vi "OpenScan LabVIEW Host.vi"() -> ()   [LabVIEW 2015]
uses:
  <vilib>/FPGAPlugInAG/PXIe-7972R/niLvFpga_Open_PXIe-7972R.vi
  <vilib>/rvi/interface/common/dynamic/niFpgaDynamicAddResources.vi
  <vilib>/FPGAPlugInAG/Dynamic/niLvFpga_Reset_Dynamic.vi
  <vilib>/FPGAPlugInAG/Dynamic/niLvFpga_Run_Dynamic.vi
  <vilib>/Utility/error.llb/Error Cluster From Error Code.vi
  <vilib>/rvi/errors/niLvFpgaAdjustHostInterfaceError.vi
  <vilib>/rvi/interface/nirviOpenFPGA/nirviOpenFPGA.xnode
  FPGA Bitfiles/OpenScan_FPGATarget_OpenScanFPGAHost_IYDpsE60iho.lvbitx
  OpenScan LabVIEW FPGA/OpenScan FPGA Host.vi
  <vilib>/rvi/interface/nirviMethod/nirviMethod.xnode
  <vilib>/rvi/interface/nirviReadWriteControl/nirviReadWriteControl.xnode
  <vilib>/rvi/interface/Simulation/niFpgaSimulationCallBeginRW.vi
  NiFpgaLv.dll
  <vilib>/rvi/errors/niLvFpgaMergeErrorWithErrorCode.vi
  <vilib>/FPGAPlugInAG/Dynamic/niLvFpga_ReadFifo_Dynamic.vi
  <vilib>/FPGAPlugInAG/Dynamic/niLvFpga_WriteFifo_Dynamic.vi
  <vilib>/FPGAPlugInAG/Dynamic/niLvFpga_StopFifo_Dynamic.vi
panel:
  out "error out":errorcluster
  out "Frame Galvo signal write done?":bool
  out "Total elements 2":u32
  out "Get status":bool=TRUE
  out "max addr":u32
  out "Ready to scan":bool
  out "Ready to initialize FPGA":bool
  in  "Filter gain":fxp<+,16,0>=0.9999847412109375 format="%.16g"
  out "Kalman done":u32
  out "Kalman done?":bool
  out "Galvo Y":u16[][](graph)
  out "Galvo X":u16[][](graph)
  out "Frames done":i32
  out "Original Image":T1(plugin-control)
  out "Kalman averaged image":T1(plugin-control)
  out "Blank image data":u32[](array[numeric])
  out "Averaged image displayed?":bool
  in  "Kalman averaging factor":u32=1
  in  "Num of frames":i32=214758367
  in  "Imaging mode":i16(ring)=2 items=["Grab, single frame", "Loop, finite frames", "Focus, infinite frames"]
  in  "Pixel clock_pulse width ratio":dbl=0.8 format="%#_13g"
  in  "Scan rate":dbl=0.25 format="%#_13g"
  in  "ZoomY":dbl=0.8 step=0.1
  in  "Zoom X":sgl=0.8 step=0.1
  in  "Calculate parameters":bool caption="停止"
  in  "Max DRAM address":u32
  in  "Frame number":i32
  in  "Samples per frame control":u32
  in  "Frame retrace time(ms)":u32=100
  in  "Number of frames":i32
  in  "Pixel pulse_initial delay":i32=1
  in  "Pixel clock_pulse width(tick)":i32
  in  "Resolution":i32(ring)=512 items=["2048"=2048, "1024"=1024, "512"=512, "256"=256]
  in  "Num of undershoot":i32=50
  in  "Elements per line":i32=1000
  in  "Total elements":u32
  in  "Pixel time (tick)":i32
  out "Image averaging done?":bool
  out "Frame acquisition done":bool
  out "Frame waveform output done":bool
  out "Waveform written to DRAM":bool
  out "Current status":T2(ring)
  in  "stop":bool caption="停止"
  in  "Load Waveform":bool caption="元素入队列"
  in  "Start Scanning":bool caption="元素入队列"
  in  "Initialize FPGA":bool caption="停止"
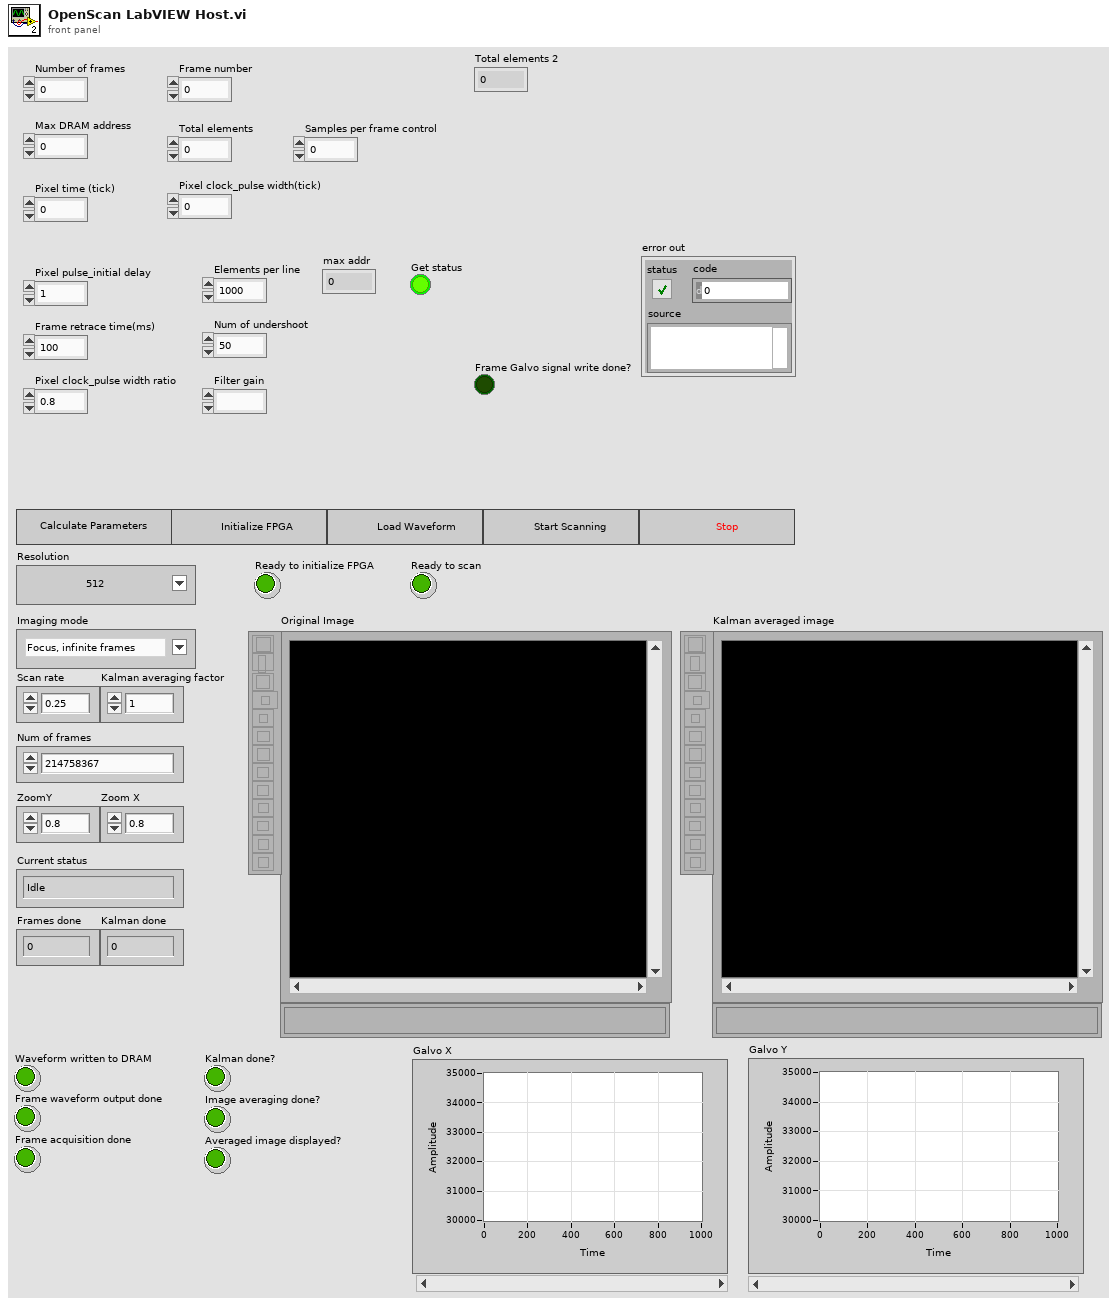
[diagram p1: front panel]
types:
  T1 = typedef "IMAQ Image.ctl" = refnum<image>
  T2 = enum16{"Idle", "Init", "Write", "Scan", "Blank", "Stop"}
  T3 = enum8{"Enabled", "Disabled", "Disabled and Grayed Out"}
  T4 = typedef "Image Type" = u32
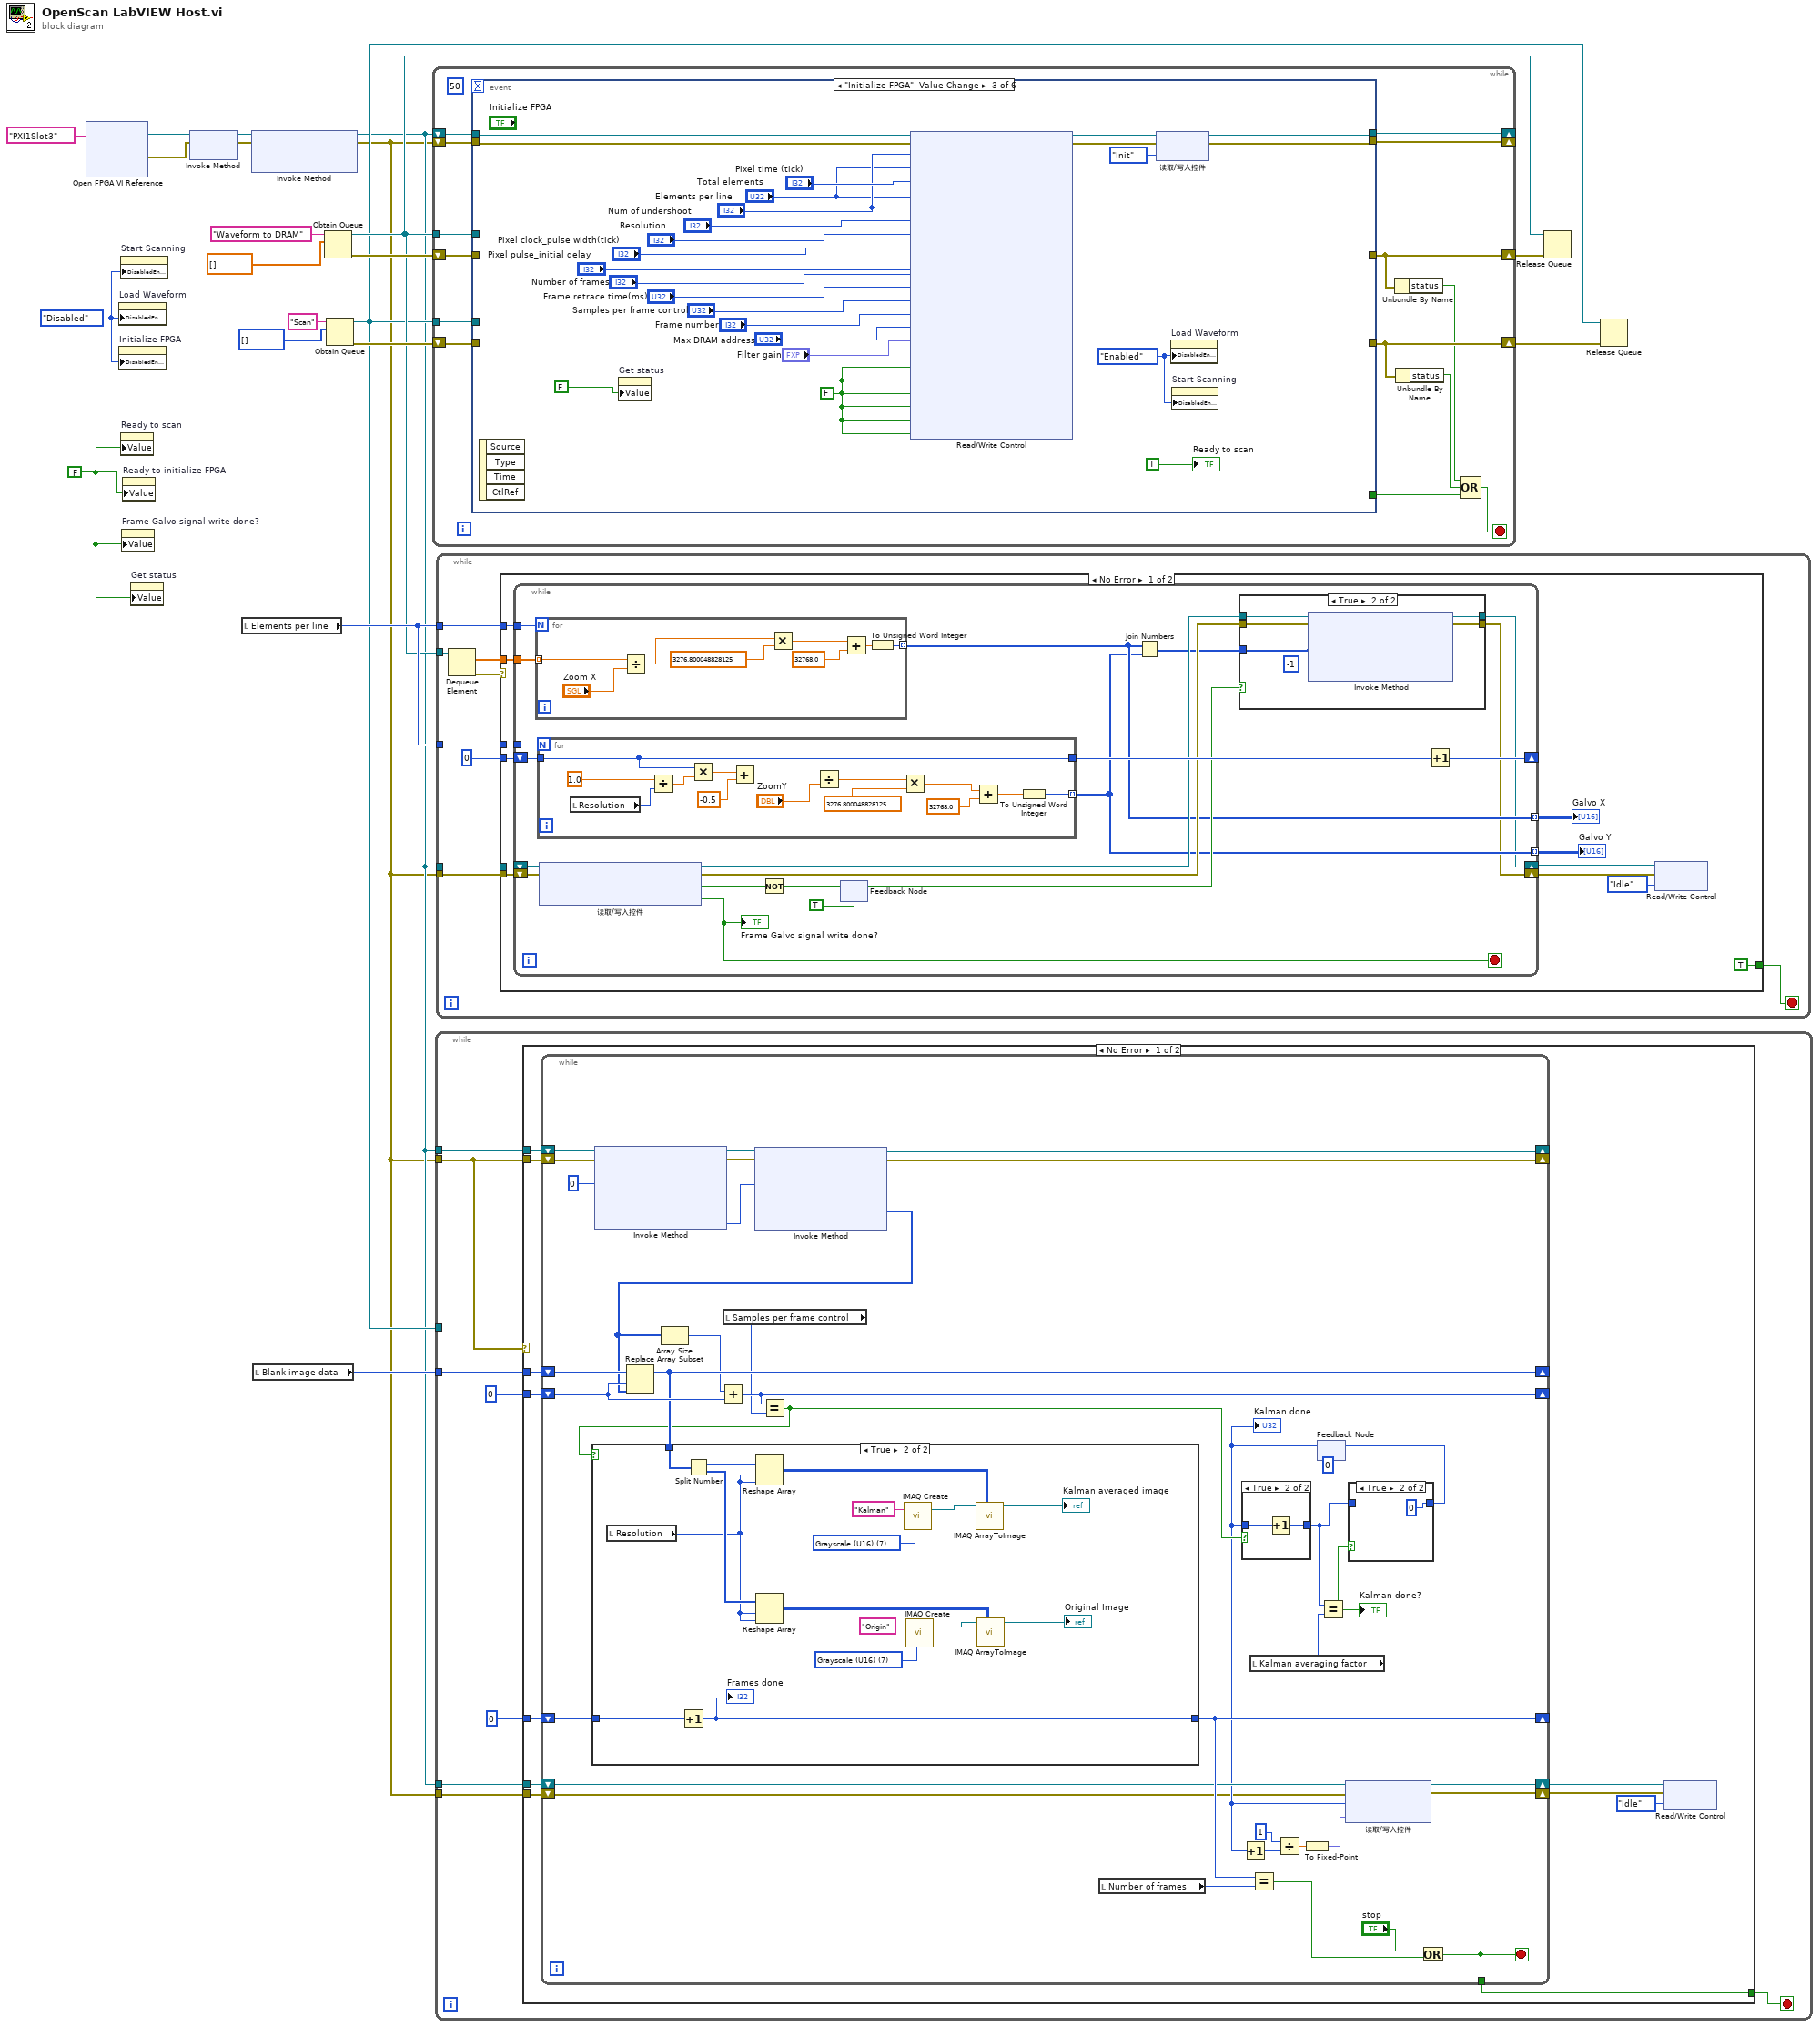
[diagram p0: block diagram]
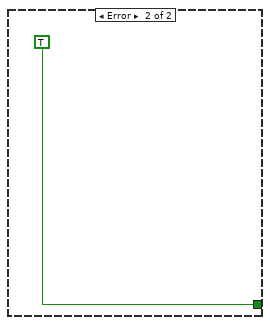
[diagram p5: hidden frame]
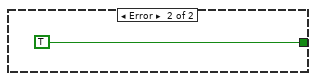
[diagram p7: hidden frame]
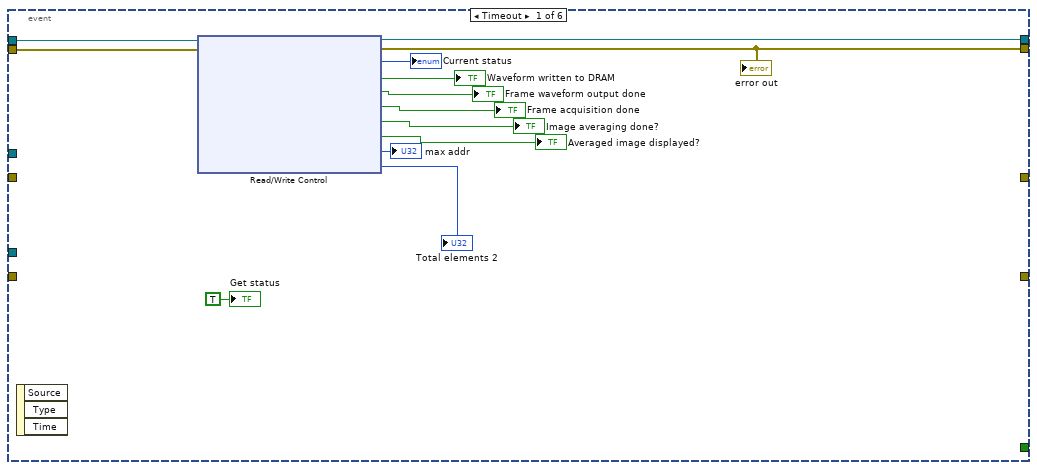
[diagram p8: hidden frame]
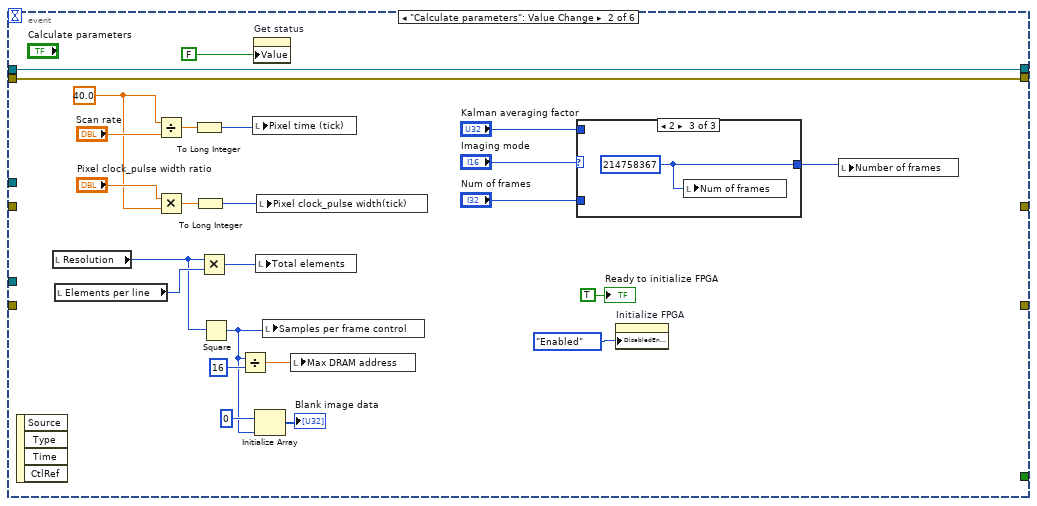
[diagram p9: hidden frame]
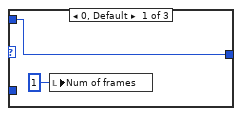
[diagram p10: hidden frame]
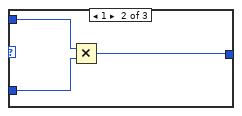
[diagram p11: hidden frame]
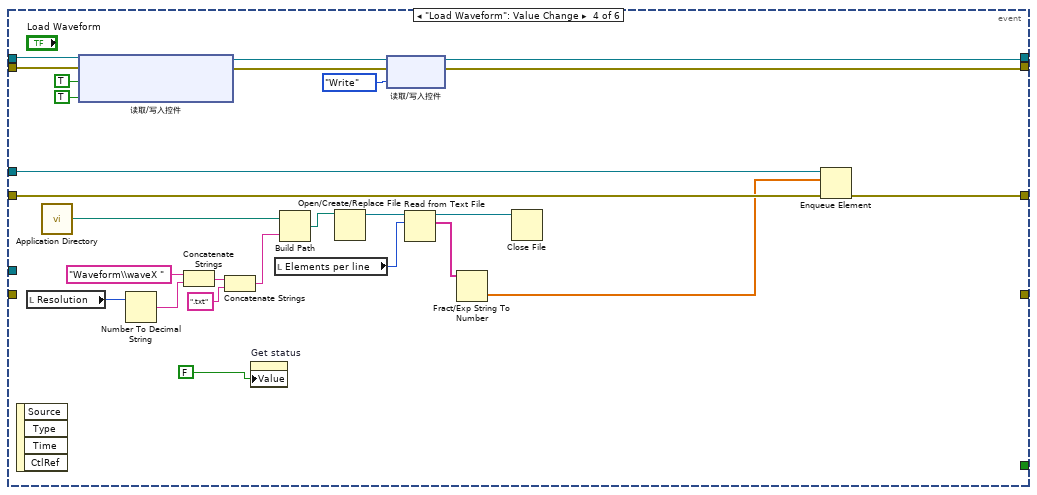
[diagram p12: hidden frame]
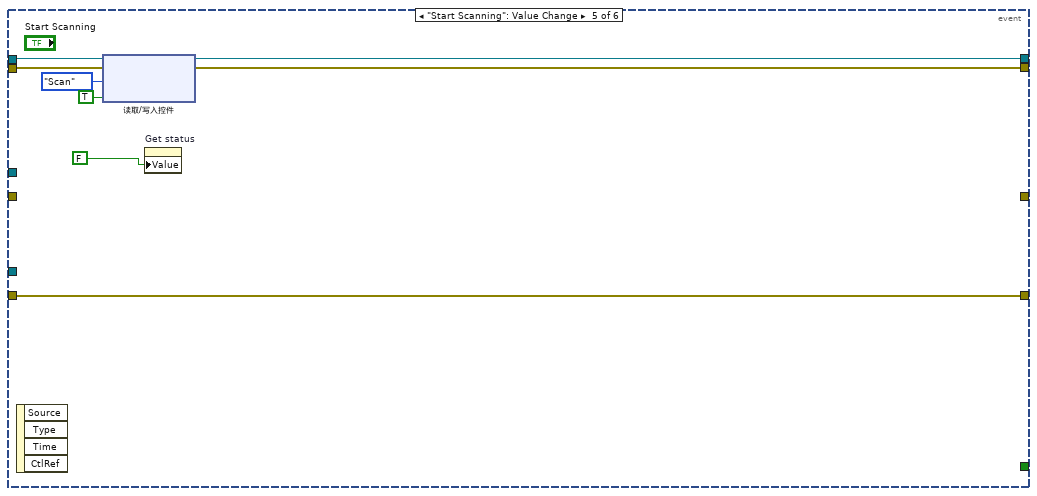
[diagram p13: hidden frame]
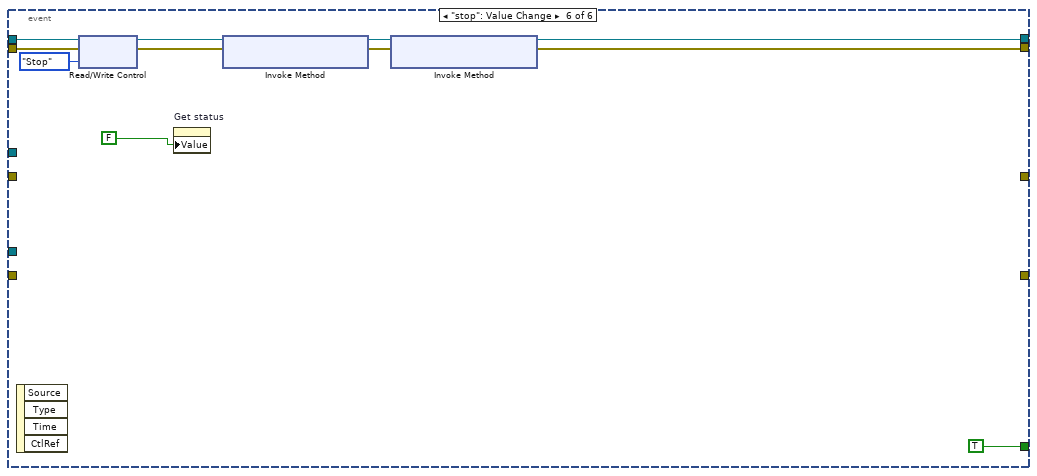
[diagram p14: hidden frame]
diagram:
  w1 = FALSE
  w4 = T3."Disabled" ("禁用")
  n1 = xnode "Open FPGA VI Reference"("resource name"=tag "PXI1Slot3" ("资源名称")) -> ("FPGA VI Reference Out"=w20:refnum<k20>, "error out"=w19:errorcluster)  [unwired: 1 in]
  n2 = property on="Load Waveform" class="Bool"("DisabledEnum"=w4) -> ()  [unwired: 2 in, 2 out]
  n3 = property on="Initialize FPGA" class="Bool"("DisabledEnum"=w4) -> ()  [unwired: 2 in, 2 out]
  n4 = property on="Start Scanning" class="Bool"("DisabledEnum"=w4) -> ()  [unwired: 2 in, 2 out]
  n5 = property on="Ready to scan" class="Bool (strict)"("Value"=w1) -> ()  [unwired: 2 in, 2 out]
  n6 = property on="Frame Galvo signal write done?" class="Bool (strict)"("Value"=w1) -> ()  [unwired: 2 in, 2 out]
  n7 = property on="Ready to initialize FPGA" class="Bool (strict)"("Value"=w1) -> ()  [unwired: 2 in, 2 out]
  n8 = property on="Get status" class="Bool (strict)"("Value"=w1) -> ()  [unwired: 2 in, 2 out]
  n9 = xnode "Invoke Method"("FPGA VI Reference In"=w20, "error in"=w19) -> ("FPGA VI Reference Out"=w18:refnum<k20>, "error out"=w17:errorcluster)
  n10 = local read "Elements per line"() -> (w13:i32)
  n11 = xnode "Invoke Method"("FPGA VI Reference In"=w18, "error in"=w17) -> ("FPGA VI Reference Out"=w3:refnum<k20>, "error out"=w2:errorcluster)  [unwired: 1 in]
  n12 = local read "Blank image data"() -> (w9:u32[])
  n13 = Obtain Queue(name (unnamed)="Waveform to DRAM" ("名称（未命名）"), element data type=dbl[] []) -> (queue out=w7:refnum<queue>, error out=w15:errorcluster)  [unwired: 3 in, 1 out]
  n14 = Obtain Queue(name (unnamed)="Scan" ("名称（未命名）"), element data type=u32[] [] ("数据")) -> (queue out=w6:refnum<queue>, error out=w11:errorcluster)  [unwired: 3 in, 1 out]
  n15 = while {
    shift-right: [w34] -> _
    shift-left: w2 -> [w35]
    tunnel: w7 -> [w33]
    shift-right: [w28] -> w8
    shift-left: w15 -> [w32]
    tunnel: w6 -> [w31]
    shift-right: [w27] -> w5
    shift-left: w11 -> [w30]
    shift-right: [w29] -> _
    shift-left: w3 -> [w36]
    stop <- w23 stop-if-true
    n16 = event shown="[2] \"Initialize FPGA\": Value Change" {
      selector: _ -> [_ _ _ _ _ _]
      dyn-events: _ -> [_ _ _ _ _ _]
      timeout: 50 -> [_ _ _ _ _ _]
      tunnel: w36 -> [w49 w51 w103 w129 w137 w147]
      tunnel: w35 -> [w44 w50 w102 w128 w136 w146]
      tunnel: [w43 w50 w89 w119 w131 w138] -> w34
      tunnel: w33 -> [_ _ _ w122 _ _]
      tunnel: w32 -> [_ _ _ w121 _ _]
      tunnel: [_ _ _ w120 _ _] -> w28
      tunnel: w31 -> [_ _ _ _ _ _]
      tunnel: w30 -> [_ _ _ _ w130 _]
      tunnel: [_ _ _ _ w130 _] -> w27
      tunnel: [w37 w51 w81 w104 w132 w139] -> w29
      tunnel: [_ _ _ _ _ TRUE] -> w24
      event Timeout {
        n17 = event-data() -> ()  [unwired: 1 in, 3 out]
        n18 = xnode "Read/Write Control"("FPGA VI Reference In"=w49, "error in"=w44) -> ("FPGA VI Reference Out"=w37:refnum<k20>, "error out"=w43:errorcluster, "Current"=→"Current status":T2, "Frame Galvo signal write done?"=→"Waveform written to DRAM":bool, "Frame waveform output finish?"=→"Frame waveform output done":bool, "Frame acquisition finish?"=→"Frame acquisition done":bool, "Image averaging done?"=→"Image averaging done?":bool, "Averaged image displayed?"=→"Averaged image displayed?":bool, "max addr"=→"max addr":u32, "Total elements"=→"Total elements 2":u32)
        "error out" <- w43
        "Get status" <- TRUE
      }
      event "Calculate parameters": Value Change {
        w69 = 40.0 ("y")
        n19 = event-data() -> ()  [unwired: 1 in, 4 out]
        n20 = local read "Resolution"() -> (w58:i32)
        n21 = local read "Elements per line"() -> (w66:i32)
        n22 = Divide(x=w69, y="Scan rate") -> (x/y=w72:dbl)
        n23 = Multiply(x="Pixel clock_pulse width ratio", y=w69) -> (x*y=w68:dbl)
        n24 = To Long Integer(number=w72) -> (32bit integer=w71:i32)
        n25 = To Long Integer(number=w68) -> (32bit integer=w67:i32)
        n26 = Multiply(x=w58, y=w66) -> (x*y=w65:i32)
        n27 = Square(x=w58) -> (x^2=w56:i32)
        n28 = Divide(x=w56, y=16) -> (x/y=w63:dbl)
        n29 = local write "Pixel time (tick)"(w71) -> ()
        n30 = property on="Get status" class="Bool (strict)"("Value"=FALSE) -> ()  [unwired: 2 in, 2 out]
        n31 = Initialize Array(u32 0, w56) -> (→"Blank image data":u32[])
        n32 = local write "Total elements"(w65) -> ()
        n33 = local write "Pixel clock_pulse width(tick)"(w67) -> ()
        n34 = local write "Samples per frame control"(w56) -> ()
        n35 = local write "Max DRAM address"(w63) -> ()
        n36 = case shown="2" "Imaging mode" {
          tunnel: "Num of frames" -> [_ w77 _]
          tunnel: [w74 w76 w79] -> w60
          tunnel: "Kalman averaging factor" -> [w74 w78 _]
          frame 0, Default {
            n37 = local write "Num of frames"(1) -> ()
          }
          frame 1 {
            n38 = Multiply(x=w78, y=w77) -> (x*y=w76:u32)
          }
          frame 2 {
            w79 = 214758367 ("Num of frames")
            n39 = local write "Num of frames"(w79) -> ()
          }
        }
        n40 = property on="Initialize FPGA" class="Bool"("DisabledEnum"=T3."Enabled" ("禁用")) -> ()  [unwired: 2 in, 2 out]
        n41 = local write "Number of frames"(w60) -> ()
        "Ready to initialize FPGA" <- TRUE
      }
      event "Initialize FPGA": Value Change {
        w80 = FALSE
        w83 = T3."Enabled" ("禁用")
        n42 = event-data() -> ()  [unwired: 1 in, 4 out]
        n43 = property on="Get status" class="Bool (strict)"("Value"=FALSE) -> ()  [unwired: 2 in, 2 out]
        n44 = xnode "Read/Write Control"("FPGA VI Reference In"=w103, "error in"=w102, "max addr"="Elements per line", "Num of elements"="Total elements", "Pixel time (tick)"="Pixel time (tick)", "Total elements"="Total elements", "Elements per line"="Elements per line", "Num of undershoot"="Num of undershoot", "Resolution"="Resolution", "Pixel clock_pulse width(tick)"="Pixel clock_pulse width(tick)", "Pixel pulse_initial delay"="Pixel pulse_initial delay", "Number of frames"="Number of frames", "Frame retrace time"="Frame retrace time(ms)", "Samples per frame control"="Samples per frame control", "Frame number"="Frame number", "Max DRAM address"="Max DRAM address", "Filter gain"="Filter gain", "Image averaging done?"=w80, "Averaged image displayed?"=w80, "Frame imaging data averaged?"=w80, "Write Frame Galvo signal?"=w80, "Write DRAM enable?"=w80, "Frame Galvo signal write done?"=w80) -> ("FPGA VI Reference Out"=w92:refnum<k20>, "error out"=w91:errorcluster)  [unwired: 1 in]
        n45 = xnode "读取/写入控件"("FPGA VI Reference In"=w92, "error in"=w91, "Current"=T2."Init") -> ("FPGA VI Reference Out"=w81:refnum<k20>, "error out"=w89:errorcluster)
        n46 = property on="Load Waveform" class="Bool"("DisabledEnum"=w83) -> ()  [unwired: 2 in, 2 out]
        n47 = property on="Start Scanning" class="Bool"("DisabledEnum"=w83) -> ()  [unwired: 2 in, 2 out]
        "Ready to scan" <- TRUE
      }
      event "Load Waveform": Value Change {
        n48 = event-data() -> ()  [unwired: 1 in, 4 out]
        n49 = local read "Resolution"() -> (w106:i32)
        n50 = call <vilib>:"Application Directory.vi"() -> ("Application Directory"=w118:path)
        n51 = xnode "读取/写入控件"("FPGA VI Reference In"=w129, "error in"=w128, "Write DRAM enable?"=TRUE, "Write Frame Galvo signal?"=TRUE) -> ("FPGA VI Reference Out"=w125:refnum<k20>, "error out"=w124:errorcluster)
        n52 = Number To Decimal String(number=w106) -> (decimal integer string=w116:string)  [unwired: 1 in]
        n53 = Concatenate Strings("Waveform\\waveX " ("名称或相对路径"), w116) -> (w115:string)
        n54 = Concatenate Strings(w115, ".txt" ("字符串")) -> (w113:string)
        n55 = property on="Get status" class="Bool (strict)"("Value"=FALSE) -> ()  [unwired: 2 in, 2 out]
        n56 = local read "Elements per line"() -> (w108:i32)
        n57 = Build Path(base path=w118, name or relative path=w113) -> (appended path=w112:path)
        n58 = Open/Create/Replace File(file path (use dialog)=w112) -> (refnum out=w111:refnum<file>)  [unwired: 5 in, 2 out]
        n59 = xnode "读取/写入控件"("FPGA VI Reference In"=w125, "error in"=w124, "Current"=T2."Write") -> ("FPGA VI Reference Out"=w104:refnum<k20>, "error out"=w119:errorcluster)
        n60 = Read from Text File(file (use dialog)=w111, count=w108) -> (refnum out=w110:refnum<file>, text=w109:string[])  [unwired: 2 in, 2 out]
        n61 = Fract/Exp String To Number(string=w109) -> (number=w107:dbl[])  [unwired: 3 in, 1 out]
        n62 = Close File(refnum=w110) -> ()  [unwired: 1 in, 2 out]
        n63 = Enqueue Element(queue=w122, element=w107, error in (no error)=w121) -> (error out=w120:errorcluster)  [unwired: 1 in, 2 out]
      }
      event "Start Scanning": Value Change {
        n64 = event-data() -> ()  [unwired: 1 in, 4 out]
        n65 = xnode "读取/写入控件"("FPGA VI Reference In"=w137, "error in"=w136, "Current"=T2."Scan", "Ready to Scan"=TRUE) -> ("FPGA VI Reference Out"=w132:refnum<k20>, "error out"=w131:errorcluster)
        n66 = property on="Get status" class="Bool (strict)"("Value"=FALSE) -> ()  [unwired: 2 in, 2 out]
      }
      event "stop": Value Change {
        n67 = event-data() -> ()  [unwired: 1 in, 4 out]
        n68 = xnode "Read/Write Control"("FPGA VI Reference In"=w147, "error in"=w146, "Current"=T2."Stop") -> ("FPGA VI Reference Out"=w143:refnum<k20>, "error out"=w142:errorcluster)
        n69 = property on="Get status" class="Bool (strict)"("Value"=FALSE) -> ()  [unwired: 2 in, 2 out]
        n70 = xnode "Invoke Method"("FPGA VI Reference In"=w143, "error in"=w142) -> ("FPGA VI Reference Out"=w141:refnum<k20>, "error out"=w140:errorcluster)
        n71 = xnode "Invoke Method"("FPGA VI Reference In"=w141, "error in"=w140) -> ("FPGA VI Reference Out"=w139:refnum<k20>, "error out"=w138:errorcluster)
      }
    }
    n72 = Unbundle By Name(w28) -> ("status"=w26:bool)
    n73 = Unbundle By Name(w27) -> ("status"=w25:bool)
    n74 = Compound Arithmetic op=OR ("复合运算")(w26, w25, w24) -> (w23:bool)
  }
  n75 = while {
    tunnel: w9 -> [w156]
    tunnel: w6 -> [_]
    tunnel: w3 -> [w153]
    tunnel: w2 -> [w150]
    tunnel: w3 -> [w151]
    tunnel: w2 -> [w149]
    stop <- w152 stop-if-true
    n76 = case shown="No Error" w149 {
      tunnel: w156 -> [w167 _]
      tunnel: 0 ("索引") -> [w166 _]
      tunnel: 0 ("索引") -> [w165 _]
      tunnel: w153 -> [w164 _]
      tunnel: [w157 TRUE] -> w152
      tunnel: w151 -> [w163 _]
      tunnel: w149 -> [w162 _]
      tunnel: w150 -> [w161 _]
      frame No Error {
        n77 = while {
          shift-right: [w201] -> _
          shift-left: w166 -> [w202]
          shift-right: [w200] -> _
          shift-left: w167 -> [w203]
          shift-right: [w198] -> _
          shift-left: w165 -> [w199]
          shift-right: [w178] -> _
          shift-left: w163 -> [w180]
          shift-right: [w177] -> _
          shift-left: w162 -> [w176]
          shift-right: [w174] -> w160
          shift-left: w164 -> [w197]
          shift-right: [w173] -> w159
          shift-left: w161 -> [w175]
          tunnel: [w168] -> w157
          stop <- w168 stop-if-true
          n78 = xnode "Invoke Method"("FPGA VI Reference In"=w180, "error in"=w176, "Number of Elements"=u32 0) -> ("FPGA VI Reference Out"=w179:refnum<k20>, "error out"=w182:errorcluster, "Elements Remaining"=w181:u32)  [unwired: 1 in, 1 out]
          n79 = local read "Samples per frame control"() -> (w195:u32)
          n80 = xnode "Invoke Method"("FPGA VI Reference In"=w179, "error in"=w182, "Number of Elements"=w181) -> ("FPGA VI Reference Out"=w178:refnum<k20>, "error out"=w177:errorcluster, "Data"=w171:u32[])  [unwired: 1 in, 1 out]
          n81 = Replace Array Subset(array=w203, new element=w171, index=w202) -> (w200:u32[])
          n82 = Array Size(array=w171) -> (size(s)=w196:i32)
          n83 = Add(x=w196, y=w202) -> (x+y=w201:i32)
          n84 = Equal?(x=w201, y=w195) -> (x = y?=w194:bool)
          n85 = case shown="True" w194 {
            tunnel: w200 -> [_ w222]
            tunnel: w199 -> [w209 w211]
            tunnel: [w209 w210] -> w198
            frame False {
            }
            frame True {
              w216 = T4 7 items=["Grayscale (U8)", "Grayscale (I16)", "Grayscale (SGL)", "Complex (CSG)", "RGB (U32)", "HSL (U32)", "RGB (U64)", "Grayscale (U16)"] ("Image Type")
              w224 = T4 7 items=["Grayscale (U8)", "Grayscale (I16)", "Grayscale (SGL)", "Complex (CSG)", "RGB (U32)", "HSL (U32)", "RGB (U64)", "Grayscale (U16)"] ("Image Type")
              n86 = local read "Resolution"() -> (w217:i32)
              n87 = Increment(x=w211) -> (x+1=w210:i32)
              "Frames done" <- w210
              n88 = Split Number(x=w222) -> (hi(x)=w221:u16[], lo(x)=w218:u16[])
              n89 = Reshape Array(w221, w217, w217) -> (w220:u16[][])
              n90 = Reshape Array(w218, w217, w217) -> (w214:u16[][])
              n91 = call "IMAQ Create"("Image Name"="Kalman", "Image Type"=w224) -> ("New Image"=w223:T1)  [unwired: 3 in, 1 out]
              n92 = call "IMAQ Create"("Image Name"="Origin", "Image Type"=w216) -> ("New Image"=w213:T1)  [unwired: 3 in, 1 out]
              n93 = call "IMAQ ArrayToImage"("Image Pixels (U16)"=w220, "Image"=w223) -> ("Image Out"=→"Kalman averaged image":T1)  [unwired: 8 in, 1 out]
              n94 = call "IMAQ ArrayToImage"("Image Pixels (U16)"=w214, "Image"=w213) -> ("Image Out"=→"Original Image":T1)  [unwired: 8 in, 1 out]
            }
          }
          n95 = local read "Number of frames"() -> (w183:i32)
          n96 = local read "Kalman averaging factor"() -> (w190:u32)
          n97 = Equal?(x=w198, y=w183) -> (x = y?=w170:bool)
          n98 = feedback #1(u32 0) -> (w188:u32)
          "Kalman done" <- w188
          n99 = case shown="True" w194 {
            tunnel: [w206 w208] -> w191
            tunnel: w188 -> [w206 w207]
            frame False {
            }
            frame True {
              n100 = Increment(x=w207) -> (x+1=w208:u32)
            }
          }
          n101 = Increment(x=w188) -> (x+1=w187:u32)
          n102 = Divide(x=u32 1, y=w187) -> (x/y=w185:dbl)
          n103 = To Fixed-Point(number=w185) -> (fixed-point=w184:fxp<+,32,0>)  [unwired: 1 in]
          n104 = Equal?(x=w191, y=w190) -> (x = y?=w189:bool)
          "Kalman done?" <- w189
          n105 = xnode "读取/写入控件"("FPGA VI Reference In"=w197, "error in"=w175, "Frame number"=w188, "Kalman gain"=w184) -> ("FPGA VI Reference Out"=w174:refnum<k20>, "error out"=w173:errorcluster)
          n106 = case shown="True" w189 {
            tunnel: w191 -> [w204 _]
            tunnel: [w204 u32 0] -> w193
            frame False {
            }
            frame True {
            }
          }
          n107 = feedback-in #1(w193) -> ()
          n108 = Or(x="stop", y=w170) -> (x .or. y?=w168:bool)
        }
        n109 = xnode "Read/Write Control"("FPGA VI Reference In"=w160, "error in"=w159, "Current"=T2."Idle") -> ()  [unwired: 2 out]
      }
      frame Error {
      }
    }
  }
  n110 = while {
    tunnel: w7 -> [w235]
    tunnel: w3 -> [w233]
    tunnel: w13 -> [w232]
    tunnel: w13 -> [w231]
    tunnel: w2 -> [w227]
    stop <- w228 stop-if-true
    n111 = Dequeue Element(queue=w235) -> (element=w234:dbl[], error out=w229:errorcluster)  [unwired: 2 in, 2 out]
    n112 = case shown="No Error" w229 {
      tunnel: w234 -> [w247 _]
      tunnel: w233 -> [w246 _]
      tunnel: w232 -> [w245 _]
      tunnel: w231 -> [w244 _]
      tunnel: 0 ("dimension size") -> [w243 _]
      tunnel: [TRUE TRUE] -> w228
      tunnel: w227 -> [w240 _]
      frame No Error {
        n113 = while {
          tunnel: w247 -> [w267]
          tunnel: w245 -> [w264]
          tunnel: w244 -> [w263]
          shift-right: [w261] -> _
          shift-left: w243 -> [w266]
          tunnel: [w252] -> w236 mode=indexing
          tunnel: [w251] -> w241 mode=indexing
          shift-right: [w249] -> w239
          shift-left: w246 -> [w265]
          shift-right: [w248] -> w238
          shift-left: w240 -> [w250]
          stop <- w253 stop-if-true
          n114 = for {
            N: w263 -> [_]
            tunnel: [w297] -> w252 mode=indexing
            tunnel: w267 -> [w291] mode=indexing
            n115 = Divide(x=w291, y="Zoom X") -> (x/y=w292:dbl)
            n116 = Multiply(x=w292, y=sgl 3276.8) -> (x*y=w295:dbl)
            n117 = Add(x=w295, y=sgl 32768.0) -> (x+y=w293:dbl)
            n118 = To Unsigned Word Integer(number=w293) -> (unsigned 16bit integer=w297:u16)
          }
          n119 = for {
            N: w264 -> [_]
            tunnel: [w289] -> w251 mode=indexing
            tunnel: w266 -> [w276]
            tunnel: [w276] -> w262
            n120 = local read "Resolution"() -> (w277:i32)
            n121 = Divide(x=1.0, y=w277) -> (x/y=w284:dbl)
            n122 = Multiply(x=w276, y=w284) -> (x*y=w283:dbl)
            n123 = Add(x=w283, y=-0.5) -> (x+y=w280:dbl)
            n124 = Divide(x=w280, y="ZoomY") -> (x/y=w281:dbl)
            n125 = Multiply(x=w281, y=sgl 3276.8) -> (x*y=w287:dbl)
            n126 = Add(x=w287, y=sgl 32768.0) -> (x+y=w278:dbl)
            n127 = To Unsigned Word Integer(number=w278) -> (unsigned 16bit integer=w289:u16)
          }
          n128 = xnode "读取/写入控件"("FPGA VI Reference In"=w265, "error in"=w250) -> ("FPGA VI Reference Out"=w260:refnum<k20>, "error out"=w259:errorcluster, "Write DRAM done?"=w257:bool, "Frame Galvo signal write done?"=w253:bool)
          "Frame Galvo signal write done?" <- w253
          n129 = Not(x=w257) -> (.not. x?=w256:bool)
          n130 = feedback #2(TRUE) -> (w254:bool)
          n131 = feedback-in #2(w256) -> ()
          n132 = Join Numbers(hi=w252, lo=w251) -> ((hi.lo)=w258:u32[])
          n133 = case shown="True" w254 {
            tunnel: w260 -> [w269 w275]
            tunnel: w259 -> [w268 w274]
            tunnel: w258 -> [_ w273]
            tunnel: [w269 w271] -> w249
            tunnel: [w268 w270] -> w248
            frame False {
            }
            frame True {
              n134 = xnode "Invoke Method"("FPGA VI Reference In"=w275, "error in"=w274, "Data"=w273, "Timeout (ms)"=-1 ("超时(ms)")) -> ("FPGA VI Reference Out"=w271:refnum<k20>, "error out"=w270:errorcluster)  [unwired: 1 out]
            }
          }
          n135 = Increment(x=w262) -> (x+1=w261:i32)
        }
        "Galvo X" <- w236
        "Galvo Y" <- w241
        n136 = xnode "Read/Write Control"("FPGA VI Reference In"=w239, "error in"=w238, "Current"=T2."Idle") -> ()  [unwired: 2 out]
      }
      frame Error {
      }
    }
  }
  n137 = Release Queue(queue=w7, error in (no error)=w8) -> ()  [unwired: 1 in, 3 out]
  n138 = Release Queue(queue=w6, error in (no error)=w5) -> ()  [unwired: 1 in, 3 out]
